vi "ziCheckTimeout.vi"(8 "Error In":errorcluster, 10 "Timeout Value (5000ms)":u32, 11 "current tick count (ms)":u32) -> (0 "Error Out":errorcluster, 3 "Timeout?":bool)   [LabVIEW 2009, in "Zurich Instruments LabOne.lvlib"]
uses:
  <instrlib>/Zurich Instruments LabOne/Zurich Instruments LabOne.lvlib
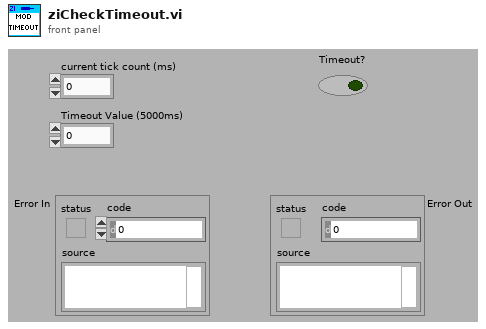
[diagram p1: front panel]
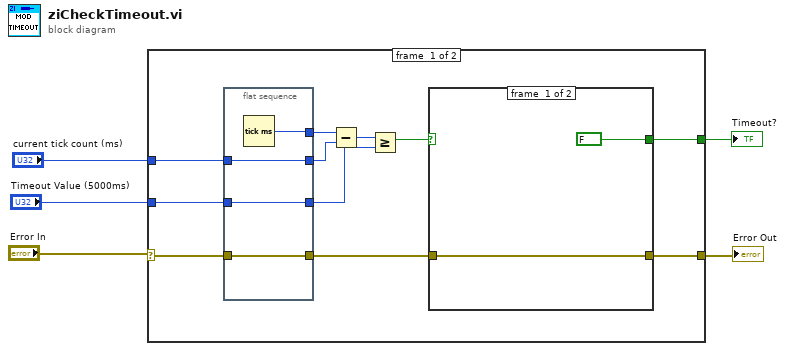
[diagram p0: block diagram]
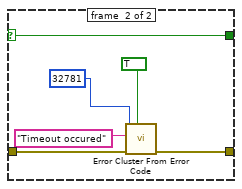
[diagram p2: hidden frame]
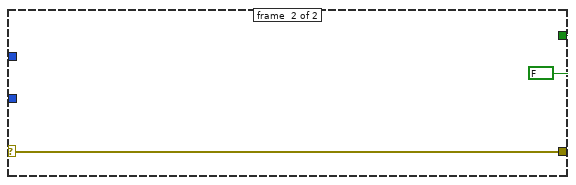
[diagram p3: hidden frame]
diagram:
  n1 = case shown="No Error" "Error In" {
    selector: "Error In" -> [w11 w30]
    tunnel: "current tick count (ms)" -> [w13 _]
    tunnel: [w9 w30] -> w3
    tunnel: "Timeout Value (5000ms)" -> [w6 _]
    tunnel: [w8 FALSE] -> w1
    frame #0 {
      n2 = flat-sequence {
        tunnel: [w20] -> w14
        tunnel: w13 -> [w19]
        tunnel: [w19] -> w12
        tunnel: w11 -> [w18]
        tunnel: [w18] -> w10
        tunnel: [w17] -> w7
        tunnel: w6 -> [w17]
        frame #0 {
          n3 = Tick Count (ms)() -> (millisecond timer value=w20:u32)
        }
      }
      n4 = Subtract(x=w14, y=w12) -> (x-y=w15:u32)
      n5 = Greater Or Equal?(x=w15, y=w7) -> (x >= y?=w16:bool)
      n6 = case shown="True" w16 {
        selector: w16 -> [_ w23]
        tunnel: w10 -> [w22 w26]
        tunnel: [w22 w25] -> w9
        tunnel: [FALSE w23] -> w8
        frame #0 {
        }
        frame #1 {
          n7 = call <vilib>:"Error Cluster From Error Code.vi"("show call chain? (False)"=TRUE, "error in (no error)"=w26, "error message (\"\")"="Timeout occured", "error code (0)"=32781) -> ("error out"=w25:errorcluster)  [unwired: 5 in]
        }
      }
    }
    frame #1 {
    }
  }
  "Error Out" <- w3
  "Timeout?" <- w1
